vi "DMSC.kill_process.vi"(1 "PID":i32, 5 "error in (no error)":errorcluster) -> (19 "error out":errorcluster)   [LabVIEW 2014, in "DMSClient.lvlib"]
doc: "kills a process"
uses:
  DMSClient.lvlib
  CSlibraries-extern/DimLVEvent/NodeMon-LV/LVNodeInfo/LVNodeInfo.lvlib
  DomainManagementUtils/DMSUtils.lvlib
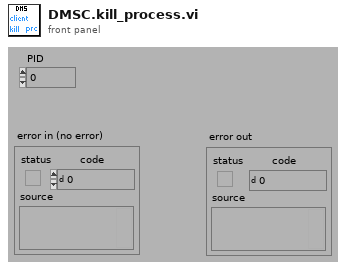
[diagram p1: front panel]
types:
  T1 = enum16{"AddMessage", "AddErrorMessage", "GetMessages"}
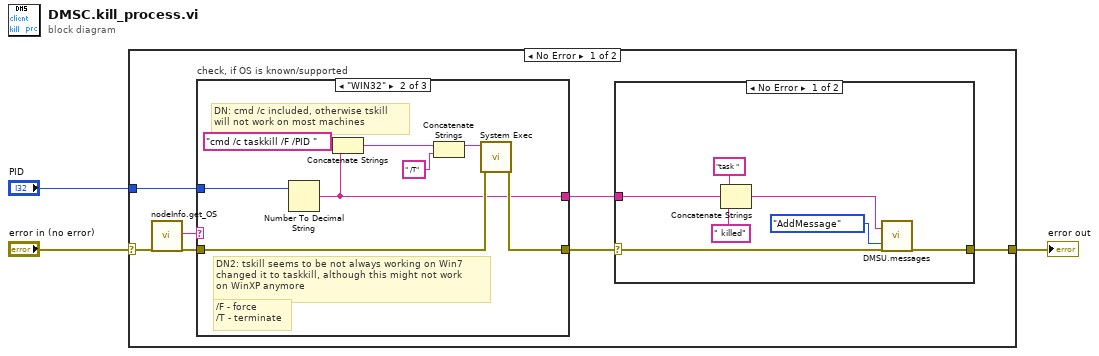
[diagram p0: block diagram]
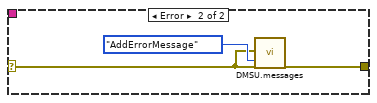
[diagram p2: hidden frame]
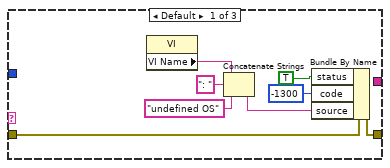
[diagram p3: hidden frame]
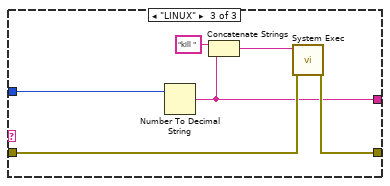
[diagram p4: hidden frame]
diagram:
  n1 = case shown="No Error" "error in (no error)" {
    selector: "error in (no error)" -> [w5 w43]
    tunnel: [w6 w43] -> w2
    tunnel: "PID" -> [w9 _]
    frame No Error {
      n2 = call "nodeInfo.get_OS.vi"("error in (no error)"=w5) -> ("OS"=w10:string, "error out"=w4:errorcluster)  [unwired: 17 in]
      n3 = case "check, if OS is known/supported" shown="\"WIN32\"" w10 {
        tunnel: w9 -> [_ w35 w42]
        tunnel: w4 -> [w21 w34 w40]
        tunnel: [w22 w33 w39] -> w8
        tunnel: [_ w32 w38] -> w7
        frame Default {
          n4 = property on="Property Node" class="VI"() -> ("VI Name"=w26:string)  [unwired: 2 in, 2 out]
          n5 = Concatenate Strings(w26, ": " ("string"), "undefined OS" ("string")) -> (w23:string)
          n6 = Bundle By Name(cluster=w21, "status"=TRUE, "code"=-1300, "source"=w23) -> (w22:errorcluster)
        }
        frame "WIN32" {
          # "/F - force\n/T - terminate"
          # "DN2: tskill seems to be not always working on Win7\nchanged it to taskkill, although this might not work \non WinXP anymore"
          # "DN: cmd /c included, otherwise tskill\nwill not work on most machines"
          n7 = Number To Decimal String(number=w35) -> (decimal integer string=w32:string)  [unwired: 1 in]
          n8 = Concatenate Strings("cmd /c taskkill /F /PID " ("string"), w32) -> (w31:string)
          n9 = Concatenate Strings(w31, " /T" ("string")) -> (w30:string)
          n10 = call <vilib>:"System Exec.vi"("error in (no error)"=w34, "command line"=w30) -> ("error out"=w33:errorcluster)  [unwired: 6 in, 3 out]
        }
        frame "LINUX" {
          n11 = Number To Decimal String(number=w42) -> (decimal integer string=w38:string)  [unwired: 1 in]
          n12 = Concatenate Strings("kill " ("string"), w38) -> (w41:string)
          n13 = call <vilib>:"System Exec.vi"("error in (no error)"=w40, "command line"=w41) -> ("error out"=w39:errorcluster)  [unwired: 6 in, 3 out]
        }
      }
      n14 = case shown="No Error" w8 {
        selector: w8 -> [w13 w19]
        tunnel: [w12 w18] -> w6
        tunnel: w7 -> [w15 _]
        frame No Error {
          n15 = Concatenate Strings("task " ("string"), w15, " killed" ("string")) -> (w11:string)
          n16 = call "DMSU.messages.vi"("message"=w11, "Action"=T1."AddMessage", "error in (no error)"=w13) -> ("error out"=w12:errorcluster)  [unwired: 15 in, 1 out]
        }
        frame Error {
          n17 = call "DMSU.messages.vi"("errorMessage"=w19, "Action"=T1."AddErrorMessage", "error in (no error)"=w19) -> ("error out"=w18:errorcluster)  [unwired: 15 in, 1 out]
        }
      }
    }
    frame Error {
    }
  }
  "error out" <- w2
